vi "SCPI_Ver.vi"(8 "error in":errorcluster, 11 "VISA in":refnum<visa-resource-name>) -> (0 "error out":errorcluster, 1 "Read":string, 2 "Timeout?":bool, 3 "VISA out":refnum<visa-resource-name>, 5 "ExecTime (ms)":i32)   [LabVIEW 2016, in "Serial_G.lvlib"]
doc: "Get SCPI version"
uses:
  Serial_G.lvlib
panel:
  # "---> Cmd to Write <---\nSYST:VERS?"
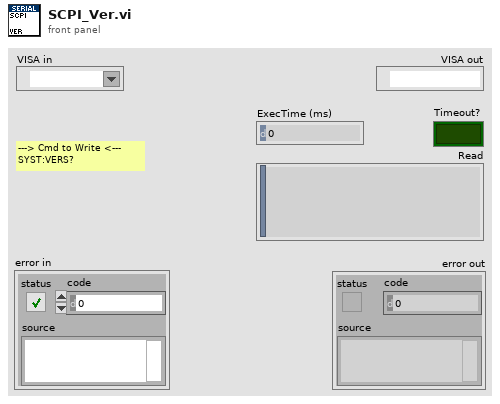
[diagram p1: front panel]
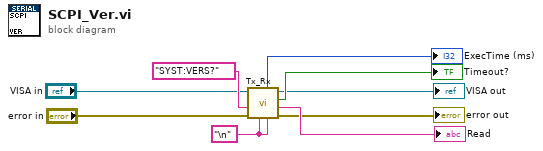
[diagram p0: block diagram]
diagram:
  w5 = "\n" ("TermChar (\\n)")
  n1 = call "Tx_Rx.vi"("Wait for? (\\n)"=w5, "TermChar (\\n)"=w5, "error in"="error in", "Write"="SYST:VERS?", "VISA in"="VISA in") -> ("error out"=→"error out":errorcluster, "Read"=→"Read":string, "Timeout?"=→"Timeout?":bool, "VISA out"=→"VISA out":refnum<visa-resource-name>, "ExecTime (ms)"=→"ExecTime (ms)":i32)  [unwired: 2 in]
